vi "Loop Async.vi"(11 "RemoteDataService in":refnum<class "RemoteDataService.lvclass">) -> ()   [LabVIEW 2020, in "Vecto.lvlib" / "RemoteDataService.lvclass"]
uses:
  RemoteDataService.lvclass
  Packet.ctl
  lv-protoc/LV-Proto/Message/Message.lvclass
  RemoteDataService.lvclass/RemoteDataService.ctl
  Timestamp ms.vi
  GroupNamesValue/GroupNamesValue.lvclass
  C:/dev/lv20CE/relink/lv-promises/Promises/Value/Value.lvclass
  SequenceCountService/Next.vi
  proto/UdpPayload/Flatten.vi
  Vecto.lvlib
  lv-promises/Promises/Promise/Promise.lvclass
panel:
  out "Proc":i32(graph)
  out "Chart":i32(graph)
  out "Local Port":u16
  out "Bind Port":u16
  out "Bind Address":u32
  out "Node ID":u32
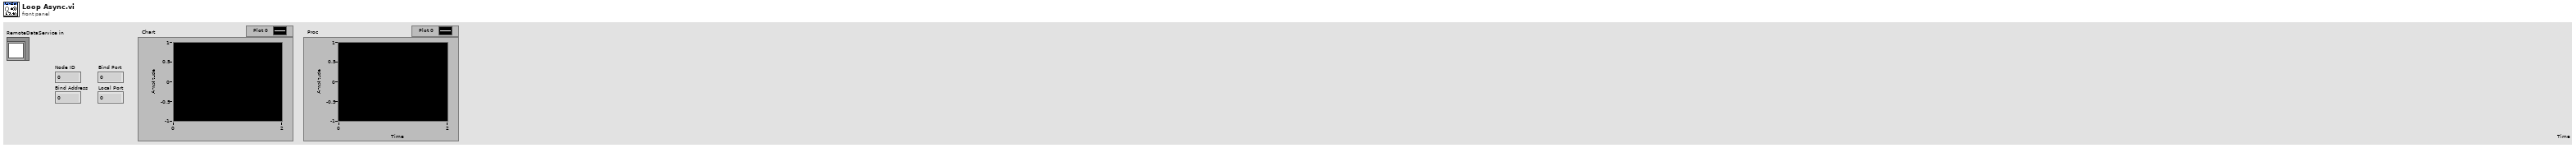
[diagram p1: front panel]
types:
  T1 = typedef "Vecto.lvlib/RemoteDataService.lvclass/Packet.ctl" = cluster{"UDP":refnum<k16>, "IP":u32, "Port":u16, "Message":refnum<class "Message.lvclass">}
  T2 = typedef "Vecto.lvlib/RemoteDataService.lvclass/Loop Data.ctl" = cluster{"Group Map":map{string, T3}, "UDP":refnum<k16>, "SequenceCountService":refnum<class "SequenceCountService.lvclass">, "Node ID":u32, "Bind Address":u32, "Bind Port":u16, "Local Port":u16, "TX Q":refnum<queue>, "Subscriptions":map{T4, T5}, "ChannelService":refnum<class "ChannelService.lvclass">}
  T3 = typedef "Vecto.lvlib/RemoteDataService.lvclass/Published Group.ctl" = cluster{"Last Publish":dbl, "Publish Address":u32, "Publish Port":u16}
  T4 = typedef "Vecto.lvlib/RemoteDataService.lvclass/Subscription.ctl" = cluster{"Multicast Address":string, "Multicast Port":u16}
  T5 = typedef "Vecto.lvlib/RemoteDataService.lvclass/Subscription Info.ctl" = cluster{"Close":refnum<user-event>}
  T6 = typedef "Vecto.lvlib/RemoteDataService.lvclass/Publish Group Data.ctl" = cluster{"GroupData":refnum<class "Msg.lvclass">}
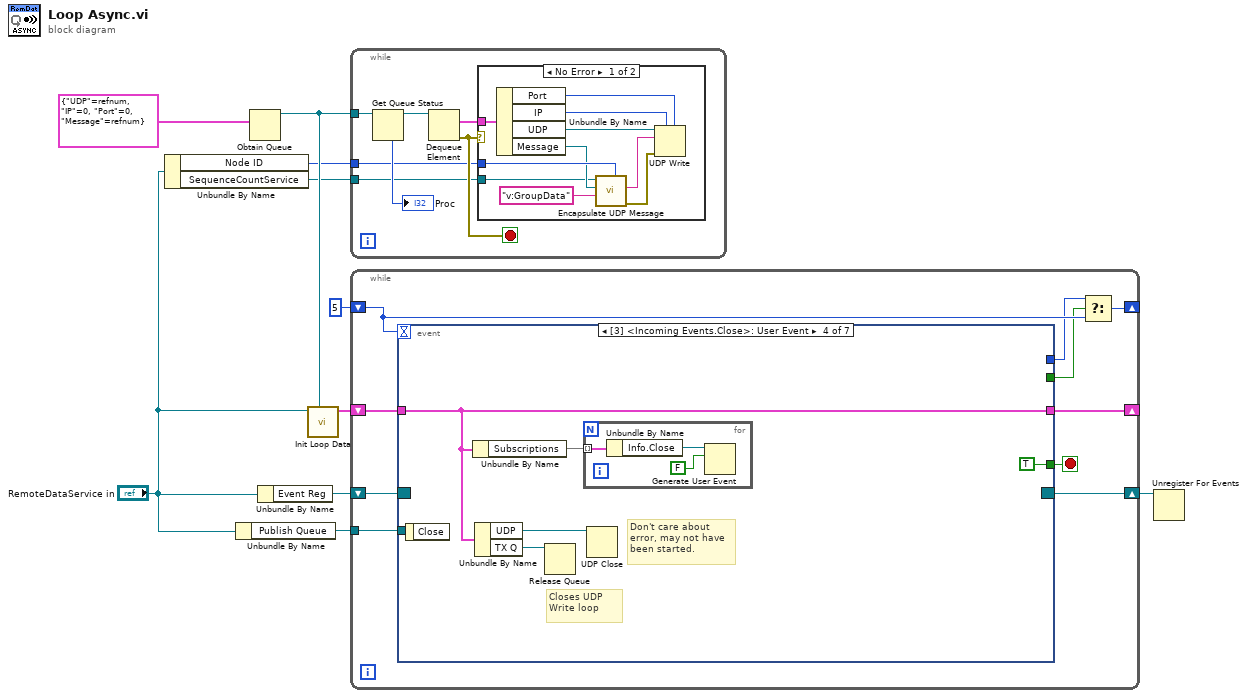
[diagram p0: block diagram]
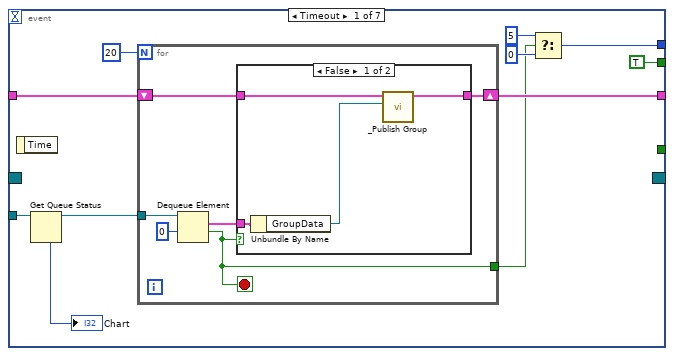
[diagram p3: hidden frame]
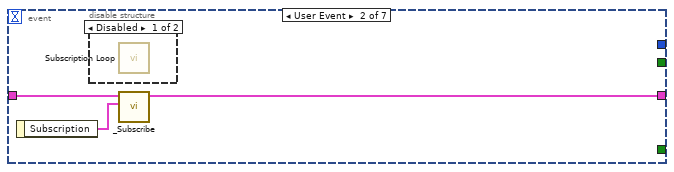
[diagram p5: hidden frame]
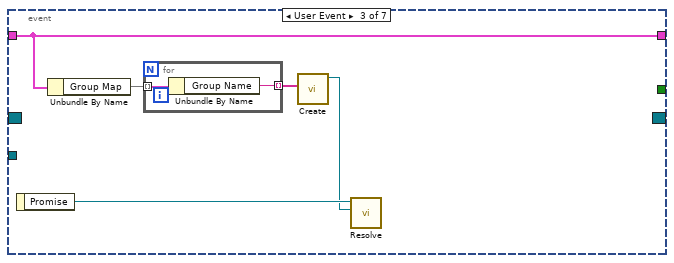
[diagram p7: hidden frame]
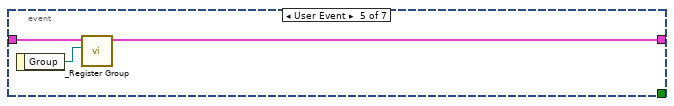
[diagram p8: hidden frame]
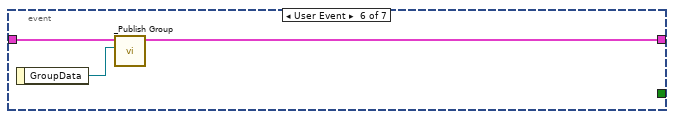
[diagram p9: hidden frame]
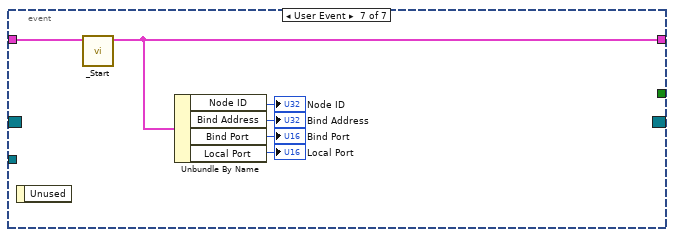
[diagram p10: hidden frame]
diagram:
  n1 = Unbundle By Name("RemoteDataService in") -> ("Node ID"=w3:u32, "SequenceCountService"=w2:refnum<class "SequenceCountService.lvclass">)
  n2 = Unbundle By Name("RemoteDataService in") -> ("Publish Queue"=w7:refnum<queue>)
  n3 = Obtain Queue(element data type=T1 {"UDP"=refnum, "IP"=0, "Port"=0, "Message"=refnum} ("Packet")) -> (queue out=w5:refnum<queue>)  [unwired: 4 in, 2 out]
  n4 = Unbundle By Name("RemoteDataService in") -> ("Event Reg"=w10:refnum<event-registration>)
  n5 = call "Init Loop Data.vi"("TX Q"=w5, "RemoteDataService in"="RemoteDataService in") -> ("Loop Data"=w8:T2)  [unwired: 9 in]
  n6 = while {
    tunnel: w5 -> [w17]
    tunnel: w3 -> [w12]
    tunnel: w2 -> [w11]
    stop <- w15 stop-if-true
    n7 = Get Queue Status(queue=w17) -> (queue out=w14:refnum<queue>, # elements in queue=→"Proc":i32)  [unwired: 2 in, 6 out]
    n8 = Dequeue Element(queue=w14) -> (element=w16:T1, error out=w15:errorcluster)  [unwired: 2 in, 2 out]
    n9 = case shown="No Error" w15 {
      tunnel: w16 -> [w27 _]
      tunnel: w12 -> [w23 _]
      tunnel: w11 -> [w21 _]
      frame No Error {
        n10 = Unbundle By Name(w27) -> ("Port"=w24:u16, "IP"=w25:u32, "UDP"=w26:refnum<k16>, "Message"=w22:refnum<class "Message.lvclass">)
        n11 = call "Encapsulate UDP Message.vi"("source_id"=w23, "type"="v:GroupData", "Encapsulated Msg"=w22, "SequenceCountService"=w21) -> ("error out"=w19:errorcluster, "UDP Payload"=w20:string)  [unwired: 6 in]
        n12 = UDP Write(address=w25, port or service name=w24, connection ID=w26, data in=w20, 8:w19) -> ()  [unwired: 1 in, 2 out]
      }
      frame Error {
      }
    }
  }
  n13 = while {
    shift-right: [w35] -> w9
    shift-left: w10 -> [w37]
    shift-right: [w34] -> _
    shift-left: w8 -> [w36]
    tunnel: w7 -> [w32]
    shift-right: [w31] -> _
    shift-left: 5 -> [w30]
    stop <- w33 stop-if-true
    n14 = event shown="[3] <Incoming Events.Close>: User Event" {
      selector: w37 -> [_ _ _ _ _ _ _]
      dyn-events: [_ _ _ _ _ _ _] -> w35
      timeout: w30 -> [_ _ _ _ _ _ _]
      tunnel: w36 -> [w45 w62 w67 w71 w80 w83 w89]
      tunnel: [w44 w61 w67 w71 w79 w81 w88] -> w34
      tunnel: [_ _ _ TRUE _ _ _] -> w33
      tunnel: w32 -> [w48 _ _ _ _ _ _]
      tunnel: [w39 _ _ _ _ _ _] -> w29
      tunnel: [TRUE _ _ _ _ _ _] -> w28
      event Timeout {
        n15 = event-data() -> ()  [unwired: 1 in, 1 out]
        n16 = Get Queue Status(queue=w48) -> (queue out=w46:refnum<queue>, # elements in queue=→"Chart":i32)  [unwired: 2 in, 6 out]
        n17 = for {
          N: 20 -> [_]
          tunnel: w46 -> [w54]
          shift-right: [w50] -> w44
          shift-left: w45 -> [w51]
          tunnel: [w49] -> w40
          stop <- w49 stop-if-true
          n18 = Dequeue Element(queue=w54, timeout in ms (-1)=0) -> (element=w52:T6, timed out?=w49:bool)  [unwired: 1 in, 2 out]
          n19 = case shown="False" w49 {
            tunnel: w52 -> [w57 _]
            tunnel: w51 -> [w58 w59]
            tunnel: [w55 w59] -> w50
            frame False {
              n20 = Unbundle By Name(w57) -> ("GroupData"=w56:refnum<class "Msg.lvclass">)
              n21 = call "_Publish Group.vi"("GroupData"=w56, "Loop Data In"=w58) -> ("Loop Data"=w55:T2)  [unwired: 8 in, 1 out]
            }
            frame True {
            }
          }
        }
        n22 = Select(t=5, s=w40, f=0) -> (s? t:f=w39:i32)
      }
      event User Event {
        n23 = event-data() -> ("Subscription"=w60:T4)  [unwired: 1 in]
        n24 = disable-structure shown="Disabled" {
          frame Disabled {
            n25 = call "Subscription Loop.vi"() -> ()  [unwired: 12 in]
          }
          frame Enabled {
          }
        }
        n26 = call "_Subscribe.vi"("Subscription"=w60, "Loop Data In"=w62) -> ("Loop Data"=w61:T2)  [unwired: 8 in, 1 out]
      }
      event User Event {
        n27 = event-data() -> ("Promise"=w64:refnum<class "Promise.lvclass">)  [unwired: 1 in]
        n28 = Unbundle By Name(w67) -> ("Group Map"=w66:map{string, T3})
        n29 = for {
          tunnel: w66 -> [w69] mode=indexing
          tunnel: [w68] -> w65 mode=indexing
          n30 = Unbundle By Name(w69) -> ("Group Name"=w68:string)
        }
        n31 = call "Create.vi"("Groups"=w65) -> ("GroupsValue out"=w63:refnum<class "GroupNamesValue.lvclass">)  [unwired: 10 in]
        n32 = call "Resolve.vi"("Result"=w63, "Promise in"=w64) -> ()  [unwired: 8 in, 2 out]
      }
      event User Event {
        # "Closes UDP Write loop"
        # "Don't care about error, may not have been started."
        n33 = event-data() -> ()  [unwired: 1 in, 1 out]
        n34 = Unbundle By Name(w71) -> ("Subscriptions"=w70:map{T4, T5})
        n35 = Unbundle By Name(w71) -> ("UDP"=w73:refnum<k16>, "TX Q"=w72:refnum<queue>)
        n36 = Release Queue(queue=w72) -> ()  [unwired: 2 in, 3 out]
        n37 = for {
          tunnel: w70 -> [w77] mode=indexing
          n38 = Unbundle By Name(w77) -> ("Info.Close"=w76:refnum<user-event>)
          n39 = Generate User Event(user event=w76, event data cluster=FALSE ("event data")) -> ()  [unwired: 2 in, 2 out]
        }
        n40 = UDP Close(connection ID=w73) -> ()  [unwired: 1 in, 2 out]
      }
      event User Event {
        n41 = event-data() -> ("Group"=w78:refnum<class "Group.lvclass">)  [unwired: 1 in]
        n42 = call "_Register Group.vi"("Group"=w78, "Loop Data In"=w80) -> ("Loop Data"=w79:T2)  [unwired: 8 in, 1 out]
      }
      event User Event {
        n43 = event-data() -> ("GroupData"=w82:refnum<class "Msg.lvclass">)  [unwired: 1 in]
        n44 = call "_Publish Group.vi"("GroupData"=w82, "Loop Data In"=w83) -> ("Loop Data"=w81:T2)  [unwired: 8 in, 1 out]
      }
      event User Event {
        n45 = event-data() -> ()  [unwired: 1 in, 1 out]
        n46 = call "_Start.vi"("Loop Data In"=w89) -> ("Loop Data"=w88:T2)  [unwired: 9 in, 1 out]
        n47 = Unbundle By Name(w88) -> ("Node ID"=→"Node ID":u32, "Bind Address"=→"Bind Address":u32, "Bind Port"=→"Bind Port":u16, "Local Port"=→"Local Port":u16)
      }
    }
    n48 = Select(t=w29, s=w28, f=w30) -> (s? t:f=w31:i32)
  }
  n49 = Unregister For Events(event registration refnum=w9) -> ()  [unwired: 1 in, 1 out]
